vi "read4Byte Tx Rx.vi"(7 "address":u16, 8 "error in (no error)":errorcluster, 9 "id":u8, 10 "protocol_version":i32, 11 "port_num":i32) -> (0 "error out":errorcluster, 3 "function return":u32)   [LabVIEW 2022 SP3, in "dxl.lvlib"]
doc: "WINDECLSPEC uint32_t read4ByteTxRx (int port_num, int protocol_version, uint8_t id, uint16_t address);"
uses:
  dxl.lvlib
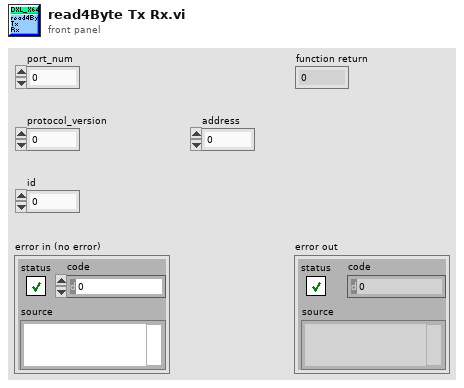
[diagram p1: front panel]
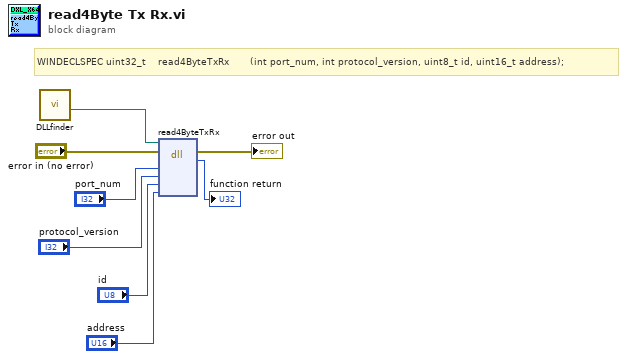
[diagram p0: block diagram]
diagram:
  # "WINDECLSPEC uint32_t    read4ByteTxRx       (int port_num, int protocol_version, uint8_t id, uint16_t address);"
  n1 = call "DLLfinder.vi"() -> ("File Path"=w1:path)  [unwired: 11 in]
  n2 = dll-call lib="C:/EnFlo Software/ADAM Serial/Instrument drivers/Dynamixel/Library/dxl_x64_c.*" fn="read4ByteTxRx"(path in=w1, error in="error in (no error)", "port_num"="port_num", "protocol_version"="protocol_version", "id"="id", "address"="address") -> (error out=→"error out":errorcluster, "return type"=→"function return":u32)  [unwired: 5 in, 1 out]
